vi "HIOKI PW3390 Conf Wiring.vi"(0 "VISA Resource":refnum<visa-resource-name>, 1 "Set/Query (F: Set)":bool, 5 "Wiring (0: 1P2W)":T1(ring), 11 "error in (no error)":errorcluster, 12 "OPC query (T: ON)":bool=TRUE, 13 "Error Out (F: Off)":bool) -> (4 "VISA Resource out":refnum<visa-resource-name>, 6 "Wiring out":T1(ring), 15 "error out":errorcluster)   [LabVIEW 2009]
doc: "Set/Query\n Set: Send the setting commands for the device.\n Query: Query the setting of the device.\n\nWiring\n Sets the wiring mode.\n\n<B>Note</B>\nThe setting for the wiring mode affects many other settings. Please set this first before starting other settings if possible.\nTo set a combination mode for multiple channels, the current sensors for the combination channels must be the same."
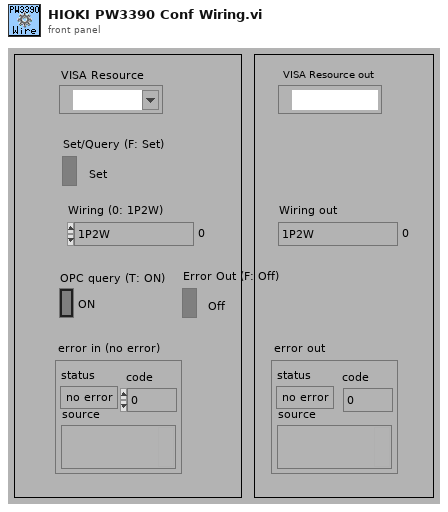
[diagram p1: front panel]
types:
  T1 = enum16{"1P2W", "1P3W, 1P2W", "3P3W2M, 1P2W", "1P3W, 1P3W", "3P3W2M, 1P3W", "3P3W2M, 3P3W2M", "3P3W3M, 1P2W", "3P4W, 1P2W"}
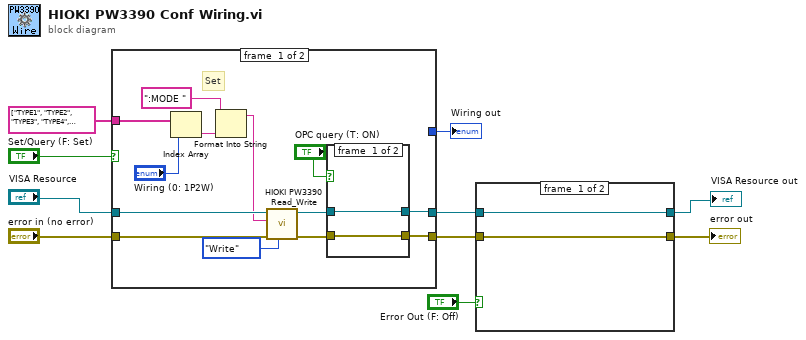
[diagram p0: block diagram]
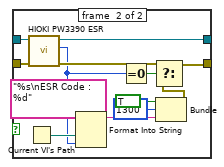
[diagram p2: hidden frame]
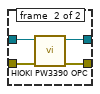
[diagram p3: hidden frame]
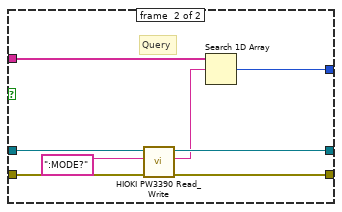
[diagram p4: hidden frame]
diagram:
  n1 = case shown="FALSE" "Set/Query (F: Set)" {
    tunnel: "error in (no error)" -> [w22 w36]
    tunnel: [w11 w33] -> w7
    tunnel: "VISA Resource" -> [w23 w35]
    tunnel: [w12 w34] -> w6
    tunnel: [_ w31] -> w4
    tunnel: string[] ["TYPE1", "TYPE2", "TYPE3", "TYPE4", "TYPE5", "TYPE6", "TYPE7", "TYPE8"] ("Strings []") -> [w18 w30]
    frame #0 {
      # "Set"
      n2 = Index Array(array=w18, index="Wiring (0: 1P2W)") -> (element=w17:string)
      n3 = Format Into String(initial string=":MODE ", w17) -> (resulting string=w20:string)  [unwired: 2 in, 1 out]
      n4 = call <instrlib>:"HIOKI PW3390 Read_Write.vi"("Read/Write"=enum16{"Read", "Write"}."Write", "error in (no error)"=w22, "data in"=w20, "VISA Resource"=w23) -> ("error out"=w13:errorcluster, "VISA Resource out"=w14:refnum<visa-resource-name>)  [unwired: 5 in, 1 out]
      n5 = case shown="TRUE" "OPC query (T: ON)" {
        tunnel: [w25 w29] -> w12
        tunnel: [w24 w28] -> w11
        tunnel: w14 -> [w25 w27]
        tunnel: w13 -> [w24 w26]
        frame #0 {
        }
        frame #1 {
          n6 = call <instrlib>:"HIOKI PW3390 OPC.vi"("error in (no error)"=w26, "VISA Resource"=w27) -> ("error out"=w28:errorcluster, "VISA Resource out"=w29:refnum<visa-resource-name>)  [unwired: 7 in, 1 out]
        }
      }
    }
    frame #1 {
      # "Query"
      n7 = call <instrlib>:"HIOKI PW3390 Read_Write.vi"("error in (no error)"=w36, "data in"=":MODE?", "VISA Resource"=w35) -> ("error out"=w33:errorcluster, "data out"=w32:string, "VISA Resource out"=w34:refnum<visa-resource-name>)  [unwired: 6 in]
      n8 = Search 1D Array(1D array=w30, element=w32) -> (index of element=w31:i32)  [unwired: 1 in]
    }
  }
  "Wiring out" <- w4
  n9 = case shown="TRUE" "Error Out (F: Off)" {
    tunnel: w6 -> [w39 w52]
    tunnel: w7 -> [w38 w51]
    tunnel: [w38 w41] -> w5
    tunnel: [w39 w50] -> w1
    frame #0 {
    }
    frame #1 {
      n10 = Current VI's Path() -> (path=w48:path)
      n11 = call <instrlib>:"HIOKI PW3390 ESR.vi"("error in (no error)"=w51, "VISA Resource"=w52) -> ("error out"=w42:errorcluster, "Output Value"=w40:u8, "VISA Resource out"=w50:refnum<visa-resource-name>)  [unwired: 6 in, 1 out]
      n12 = Format Into String(format string="%s\nESR Code : %d", w48, w40) -> (resulting string=w44:string)  [unwired: 2 in, 1 out]
      n13 = Equal To 0?(x=w40) -> (x = 0?=w49:bool)
      n14 = Bundle("status"=TRUE, "code"=1300, w44) -> (w43:cluster{"status":bool, "code":i32, string})  [unwired: 1 in]
      n15 = Select(t=w42, s=w49, f=w43) -> (s? t:f=w41:errorcluster)
    }
  }
  "error out" <- w5
  "VISA Resource out" <- w1
